vi "V_out_Spaendingsdeler.vi"(0 "AI0-PORT":tag, 4 "Antal målinger":dbl=1000.0, 9 "milliseconds to wait":u32=10) -> (14 "Kører målingerne?":bool, 19 "Volt ud":dbl)   [LabVIEW 2022 SP3]
doc: "* SPÆNDINGSDELER VOLT MÅLING *\nDenne SubVi anvender AI0+ porten til at måle spændingen i knudepunktet på spændingsdeleren.\nDette opsæt består af:\n- 1. stk 10K-Ohm modstand.\n- 1. stk NTC-Termistor.\n\nOutput kanaler på MyDAQ til målinger:\n- 5V.\n\nInput kanaler på MyDAQ til målinger:\n- AI0 +\n- AI0 -\n- AGND (& evt. GND ** Better Safe then sorry **)\n\nEt eksempel på data output:\nVolt ud: 2.467501"
uses:
  <vilib>/DAQmx/create/channels.llb/DAQmx Create Channel (AI-Voltage-Basic).vi
  <vilib>/DAQmx/read.llb/DAQmx Read (Analog DBL 1Chan 1Samp).vi
  <vilib>/Utility/error.llb/DialogType.ctl
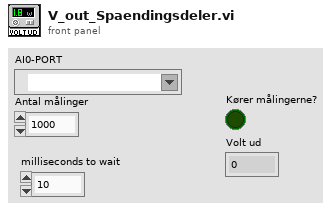
[diagram p1: front panel]
types:
  T1 = typedef "DialogType.ctl" = u16
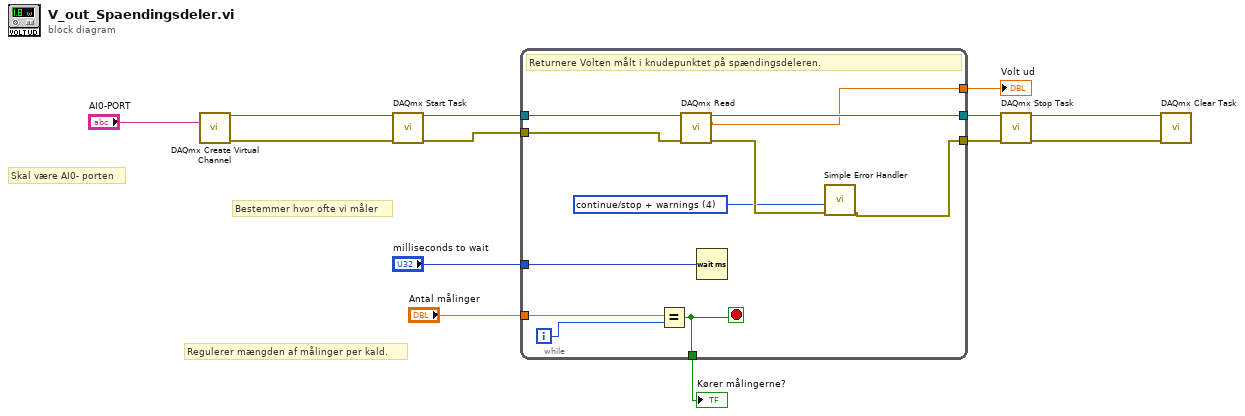
[diagram p0: block diagram]
diagram:
  # "Regulerer mængden af målinger per kald."
  # "Bestemmer hvor ofte vi måler"
  # "Skal være AI0- porten"
  n1 = call-poly <vilib>:"DAQmx Create Virtual Channel.vi"("physical channels"="AI0-PORT") -> ("task out"=w12:refnum<k21>, "error out"=w11:errorcluster)  [unwired: 13 in]
  n2 = call <vilib>:"DAQmx Start Task.vi"("task/channels in"=w12, "error in"=w11) -> ("task out"=w10:refnum<k21>, "error out"=w9:errorcluster)  [unwired: 12 in]
  n3 = while {
    tunnel: w10 -> [w24]
    tunnel: w9 -> [w23]
    tunnel: "Antal målinger" -> [w19]
    tunnel: [w18] -> w5
    tunnel: [w17] -> w4
    tunnel: [w16] -> w3
    tunnel: [w15] -> w2
    tunnel: "milliseconds to wait" -> [w14]
    i -> [w20]
    stop <- w16 stop-if-true
    w21 = T1 4 items=["no dialog", "OK message", "continue or stop message", "OK message + warnings", "continue/stop + warnings"] ("type of dialog (OK msg:1)")
    # "Returnere Volten målt i knudepunktet på spændingsdeleren."
    n4 = Equal?(x=w19, y=w20) -> (x = y?=w16:bool)
    n5 = call-poly <vilib>:"DAQmx Read.vi"("task/channels in"=w24, "error in"=w23) -> ("task out"=w18:refnum<k21>, "data"=w15:dbl, "error out"=w22:errorcluster)  [unwired: 11 in]
    n6 = Wait (ms)(milliseconds to wait=w14) -> ()  [unwired: 1 out]
    n7 = call <vilib>:"Simple Error Handler.vi"("type of dialog (OK msg:1)"=w21, "error in (no error)"=w22) -> ("error out"=w17:errorcluster)  [unwired: 3 in, 4 out]
  }
  "Volt ud" <- w2
  "Kører målingerne?" <- w3
  n8 = call <vilib>:"DAQmx Stop Task.vi"("task/channels in"=w5, "error in"=w4) -> ("task out"=w7:refnum<k21>, "error out"=w6:errorcluster)  [unwired: 12 in]
  n9 = call <vilib>:"DAQmx Clear Task.vi"("task in"=w7, "error in"=w6) -> ()  [unwired: 13 in, 1 out]
